vi "IDS_system_setIpSettings.vi"(0 "deviceHandle":i32, 1 "ipaddress":string, 2 "subnetmask":string, 3 "defaultgateway":string, 4 "setmode":i32, 5 "error in (no error)":errorcluster) -> (14 "deviceHandle out":i32, 19 "error out":errorcluster)   [LabVIEW 2016]
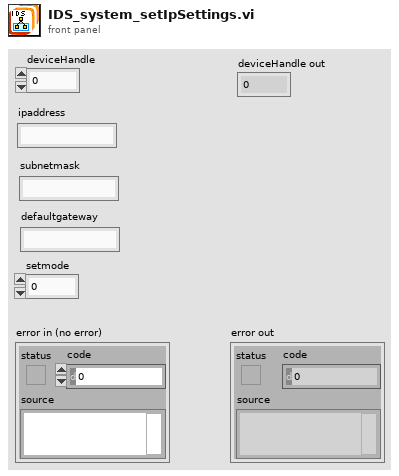
[diagram p1: front panel]
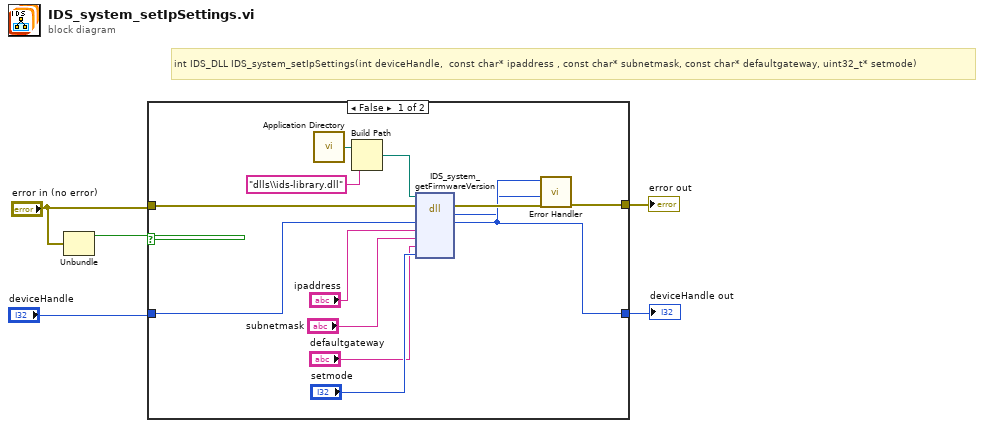
[diagram p0: block diagram]
diagram:
  # "int IDS_DLL IDS_system_setIpSettings(int deviceHandle,  const char* ipaddress , const char* subnetmask, const char* defaultgateway, uint32_t* setmode)"
  n1 = Unbundle("error in (no error)") -> ("status"=w1:bool)  [unwired: 2 out]
  n2 = case shown="False" w1 {
    tunnel: "error in (no error)" -> [w17 w20]
    tunnel: [w15 w20] -> w5
    tunnel: "deviceHandle" -> [w14 w19]
    tunnel: [w13 w19] -> w3
    frame False {
      n3 = call <vilib>:"Application Directory.vi"() -> ("Application Directory"=w8:path)
      n4 = Build Path(base path=w8, name or relative path="dlls\\ids-library.dll" ("ipAddress")) -> (appended path=w6:path)
      n5 = dll-call lib="C:/Users/matheus/Desktop/LabVIEW_Draft_V1.6.0/dlls/ids-library.*" fn="IDS_system_getFirmwareVersion"(path in=w6, error in=w17, "deviceHandle"=w14, "ipaddress"="ipaddress", "subnetmask"="subnetmask", "defaultgateway"="defaultgateway", "setmode"="setmode") -> (error out=w16:errorcluster, "Rückgabetyp"=w12:i32, "deviceHandle"=w13:i32)  [unwired: 5 in, 1 out]
      n6 = call "Error Handler.vi"("error in (no error)"=w16, "error code"=w12, "deviceHandle"=w13) -> ("error out"=w15:errorcluster)  [unwired: 7 in, 1 out]
    }
    frame True {
    }
  }
  "error out" <- w5
  "deviceHandle out" <- w3
